vi "Write CtlRange.vi"(8 "error in (no error)":errorcluster, 10 "CtlRange":cluster{"high":dbl, "low":dbl}={"high"=0.0, "low"=-5.0}, 11 "Humidity Control in":refnum<class "Humidity Control.lvclass">) -> (0 "error out":errorcluster, 3 "Humidity Control out":refnum<class "Humidity Control.lvclass">)   [LabVIEW 2012, in "Humidity Control.lvclass"]
uses:
  Humidity Control.lvclass
  Humidity Control.lvclass/Humidity Control.ctl
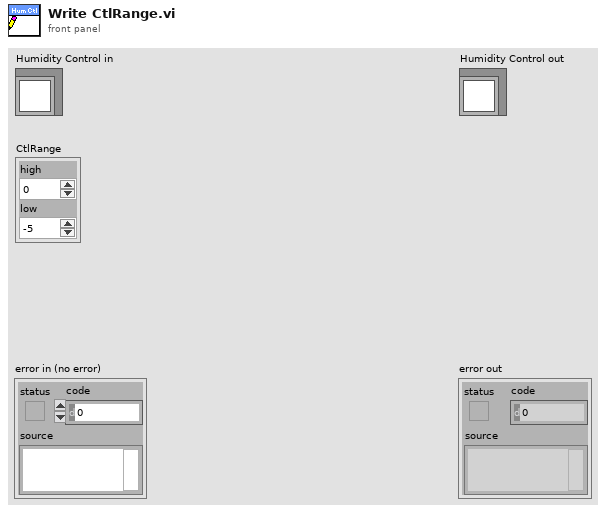
[diagram p1: front panel]
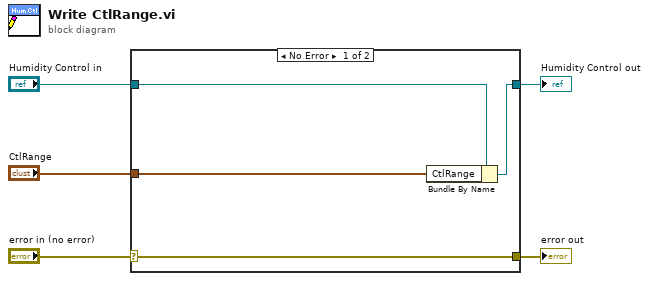
[diagram p0: block diagram]
diagram:
  n1 = case shown="No Error" "error in (no error)" {
    selector: "error in (no error)" -> [w9 w10]
    tunnel: [w9 w10] -> w4
    tunnel: [w7 w11] -> w2
    tunnel: "Humidity Control in" -> [w8 w11]
    tunnel: "CtlRange" -> [w6 _]
    frame No Error {
      n2 = Bundle By Name(cluster=w8, "CtlRange"=w6) -> (w7:refnum<class "Humidity Control.lvclass">)
    }
    frame Error {
    }
  }
  "error out" <- w4
  "Humidity Control out" <- w2
